vi "Parameter Druck Sensoren.vi"() -> ()   [LabVIEW 2020, in "Erweiterte Konfig.lvlib"]
uses:
  Erweiterte Konfig.lvlib
  Parameter Sensoren.ctl
  Visualisierungs Elemente/Button.ctl
  FGV PID Aktionen.ctl
  Passwortverwaltung/FGV Passwort Aktion.ctl
  Allgemein/Aktionen Daten am cRIO speichern.ctl
  Passwortverwaltung/Passwort.lvlib
  Allgemein/allgemeine Sub-VIs.lvlib
  cRIO/PC/Kommunikation mit cRIO.lvlib
panel:
  out "Roh Druck Kalter Block":sgl caption="V" format="%.3f"
  out "Druck Kalter Block":sgl caption="bar" format="%.2f"
  in  "speichern":T1
  in  "abbrechen":T1
  out "Roh Durck FTIR IAG":sgl caption="V" format="%.3f"
  out "Roh Durck CG":sgl caption="V" format="%.3f"
  out "Roh Druck CG PMA":sgl caption="V" format="%.3f"
  out "Roh Durchfl.PMA":sgl caption="V" format="%.3f"
  out "Roh Durck Kalt":sgl caption="V" format="%.3f"
  out "Roh Druck Ausgang":sgl caption="V" format="%.3f"
  out "Roh Durchfl.FTIR":sgl caption="V" format="%.3f"
  out "Druck FTIR IAG":sgl caption="atm" format="%.3f"
  out "Druck CG":sgl caption="bar" format="%.2f"
  out "Druck CG PMA":sgl caption="bar" format="%.2f"
  out "Druck Umgebung":sgl caption="mbar" format="%#.0f"
  out "Druck Ausgang":sgl caption="mbar" format="%#.0f"
  out "Durchfluss PMA":sgl caption="l/min" format="%.1f"
  out "Durchfluss FTIR":sgl caption="l/min" format="%.1f"
  in  "Parameter Sensoren":T2 {"Druck Kalter Block" format="%#_5g"; "Offset Druck FTIR IAG" format="%#_5g"; "Offset Druck CG" format="%#_5g"; "Offset Druck CG PMA" format="%#_5g"; "Offset Durchfl.PMA" format="%#_5g"; "Offset Druck Umgebung" format="%#_5g"; "Offset Druck Ausgang" format="%#_5g"; "Offset Durchfl.FTIR" format="%#_5g"; "Kal.Durchfl.PMA" format="%.3g"; "Kal.Durchfl.FTIR" format="%.3g"}
  # "Sensor"
  # "Istwert"
  # "Kalibrierwert"
  # "Offset"
  # "Rohwert"
  # "Durchfluss FTIR:"
  # "Druck Ausgang:"
  # "Umgebungsdruck:"
  # "Druck CG:"
  # "Druck FTIR IAG:"
  # "Flow PMA:"
  # "Pressure CG PMA:"
  # "Druck Kalter Block:"
  # "Sensor Konfiguration"
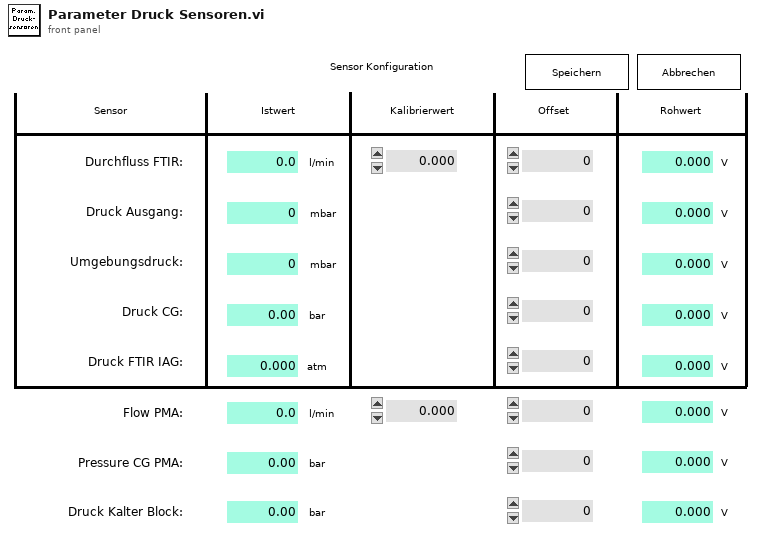
[diagram p1: front panel]
types:
  T1 = typedef "Button.ctl" = bool
  T2 = typedef "Erweiterte Konfig.lvlib/Parameter Sensoren.ctl" = cluster{"Kal.Durchfl.FTIR":sgl, "Kal.Durchfl.PMA":sgl, "Offset Durchfl.FTIR":sgl, "Offset Druck Ausgang":sgl, "Offset Druck Umgebung":sgl, "Offset Durchfl.PMA":sgl, "Offset Druck CG PMA":sgl, "Offset Druck CG":sgl, "Offset Druck FTIR IAG":sgl, "Druck Kalter Block":sgl}
  T3 = typedef "Erweiterte Konfig.lvlib/FGV PID Aktionen.ctl" = enum16{"Lesen", "Schreiben PID", "Schreiben Sonstige", "Dichtheitstest", "Aktionen Dicht.", "Parameter Sensor"}
  T4 = typedef "Passwort.lvlib/FGV Passwort Aktion.ctl" = enum16{"prüfen", "setzen", "Initialisieren", "PW speichern", "lesen", "PW Änderung"}
  T5 = typedef "allgemeine Sub-VIs.lvlib/Aktionen Daten am cRIO speichern.ctl" = enum16{"lesen", "speichern setzen", "speichern reset", "gespeichert"}
  T6 = typedef "Verwaltung - cRIO.lvlib/Analog Eingaenge.ctl" = cluster{"AI0: Durchfluss FT-IR":sgl, "AI1: Druck Ausgang":sgl, "AI2: Umgebungsdruck":sgl, "AI3: Druck FT-IR":sgl, "AI4: Druck CalGas":sgl, "AI5: Reserve":sgl, "AI6: Reserve":sgl, "AI7: Reserve":sgl, "Rohwert Durchfluss FT-IR":sgl, "Rohwert Druck Ausgang":sgl, "Rohwert Umgebungsdruck":sgl, "Rohwert Druck FT-IR":sgl, "Rohwert Druck CalGas":sgl, "Rohwert AI5":sgl, "Rohwert AI6":sgl, "Rohwert AI7":sgl, "Rohwert Diffdruck mbar FTIR":sgl}
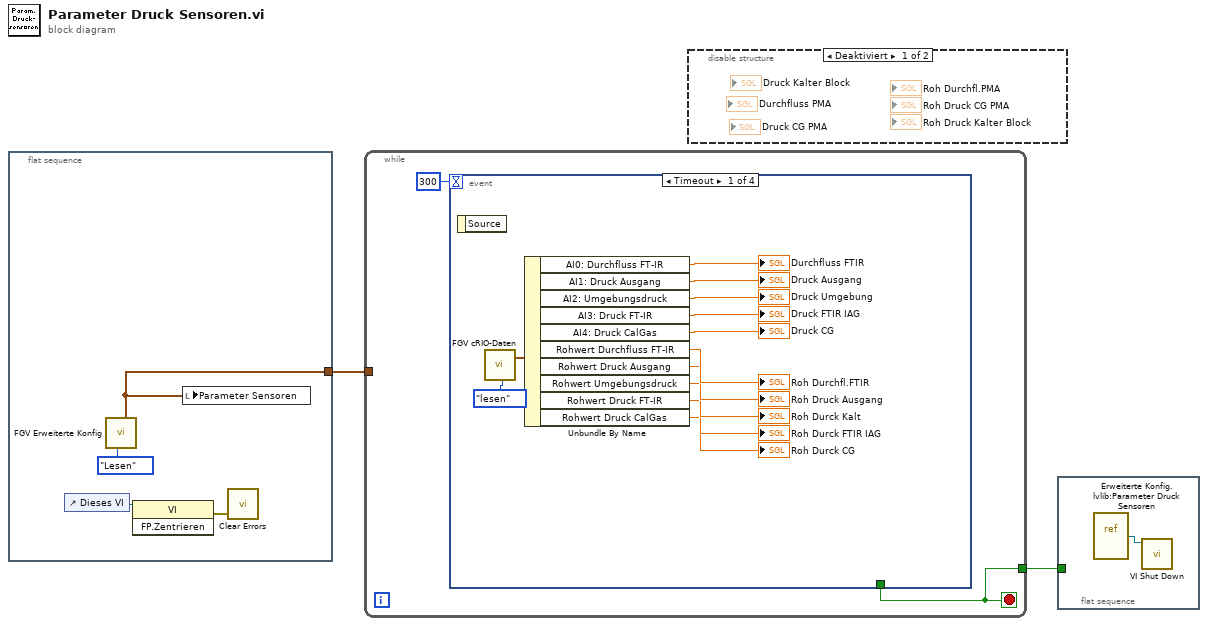
[diagram p0: block diagram]
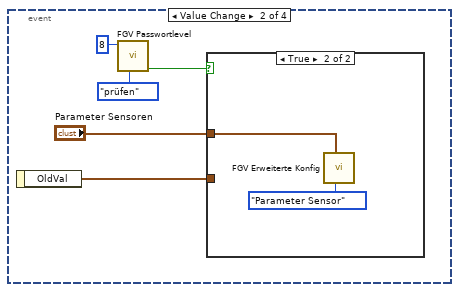
[diagram p3: hidden frame]
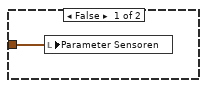
[diagram p4: hidden frame]
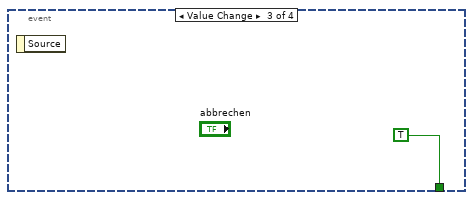
[diagram p5: hidden frame]
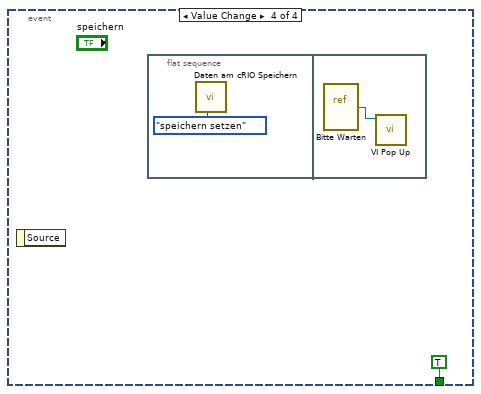
[diagram p6: hidden frame]
diagram:
  n1 = flat-sequence {
    tunnel: [w5] -> w2
    frame #0 {
      n2 = control-ref of="Dieses VI"() -> (w4:refnum<vi>)
      n3 = call "FGV Erweiterte Konfig.vi"("Aktion"=FGV_PID_Aktionen."Lesen") -> ("Parameter Sensoren"=w5:T2)  [unwired: 5 in, 5 out]
      n4 = invoke class="VI" method="FP.Zentrieren"(reference=w4) -> (error out=w3:errorcluster)  [unwired: 2 in, 2 out]
      n5 = local write "Parameter Sensoren"(w5) -> ()
      n6 = call <vilib>:"Clear Errors.vi"("error in (no error)"=w3) -> ()  [unwired: 5 in, 2 out]
    }
  }
  n7 = while {
    tunnel: w2 -> [_]
    tunnel: [w8] -> w1
    stop <- w8 stop-if-true
    n8 = event shown="[0] Timeout" {
      selector: _ -> [_ _ _ _]
      dyn-events: _ -> [_ _ _ _]
      timeout: 300 -> [_ _ _ _]
      tunnel: [_ _ TRUE ("abbrechen") TRUE ("abbrechen")] -> w8
      event Timeout {
        n9 = event-data() -> ()  [unwired: 1 in, 1 out]
        n10 = call "FGV cRIO-Daten.vi"("Aktion"=enum16{"lesen", "schreiben"}."lesen") -> ("Analog Input"=w19:T6)  [unwired: 9 in, 9 out]
        n11 = Unbundle By Name(w19) -> ("AI0: Durchfluss FT-IR"=→"Durchfluss FTIR":sgl, "AI1: Druck Ausgang"=→"Druck Ausgang":sgl, "AI2: Umgebungsdruck"=→"Druck Umgebung":sgl, "AI3: Druck FT-IR"=→"Druck FTIR IAG":sgl, "AI4: Druck CalGas"=→"Druck CG":sgl, "Rohwert Durchfluss FT-IR"=→"Roh Durchfl.FTIR":sgl, "Rohwert Druck Ausgang"=→"Roh Druck Ausgang":sgl, "Rohwert Umgebungsdruck"=→"Roh Durck Kalt":sgl, "Rohwert Druck FT-IR"=→"Roh Durck FTIR IAG":sgl, "Rohwert Druck CalGas"=→"Roh Durck CG":sgl)
      }
      event Value Change {
        n12 = event-data() -> ("OldVal"=w21:T2)  [unwired: 1 in]
        n13 = call "FGV Passwortlevel.vi"("FGV Passwort Aktion"=FGV_Passwort_Aktion."prüfen", "geforderter Level"=i16 8) -> ("Freigabe"=w23:bool)  [unwired: 7 in, 2 out]
        n14 = case shown="True" w23 {
          tunnel: "Parameter Sensoren" -> [_ w27]
          tunnel: w21 -> [w26 _]
          frame False {
            n15 = local write "Parameter Sensoren"(w26) -> ()
          }
          frame True {
            n16 = call "FGV Erweiterte Konfig.vi"("Aktion"=FGV_PID_Aktionen."Parameter Sensor", "Parameter Sensoren"=w27) -> ()  [unwired: 4 in, 6 out]
          }
        }
      }
      event Value Change {
        n17 = event-data() -> ()  [unwired: 1 in, 1 out]
      }
      event Value Change {
        n18 = event-data() -> ()  [unwired: 1 in, 1 out]
        n19 = flat-sequence {
          frame #0 {
            n20 = call "Daten am cRIO Speichern.vi"("Aktionen"=Aktionen_Daten_am_cRIO_speichern."speichern setzen") -> ()  [unwired: 9 in, 2 out]
          }
          frame #1 {
            n21 = vi-ref "Bitte Warten.vi"() -> (w32:refnum<vi>)
            n22 = call "VI Pop Up.vi"("VI Referenz"=w32) -> ()  [unwired: 10 in, 1 out]
          }
        }
      }
    }
  }
  n23 = disable-structure shown="Deaktiviert" {
    frame Disabled {
    }
    frame Enabled {
    }
  }
  n24 = flat-sequence {
    tunnel: w1 -> [_]
    frame #0 {
      n25 = vi-ref "Erweiterte Konfig.lvlib:Parameter Druck Sensoren.vi"() -> (w33:refnum<vi>)
      n26 = call "VI Shut Down.vi"("VI Referenz"=w33) -> ()  [unwired: 11 in]
    }
  }
